vi "Shut Down Device.vi"(8 "error in (no error)":errorcluster, 11 "Power Meter in":refnum<class "Power Meter.lvclass">) -> (0 "error out":errorcluster, 3 "Power Meter out":refnum<class "Power Meter.lvclass">)   [LabVIEW 2018, in "Power Meter.lvlib" / "Power Meter.lvclass"]
uses:
  Power Meter.lvclass
  Power Meter.lvclass/Power Meter.ctl
  Device/Device.lvclass
  Power Meter.lvlib
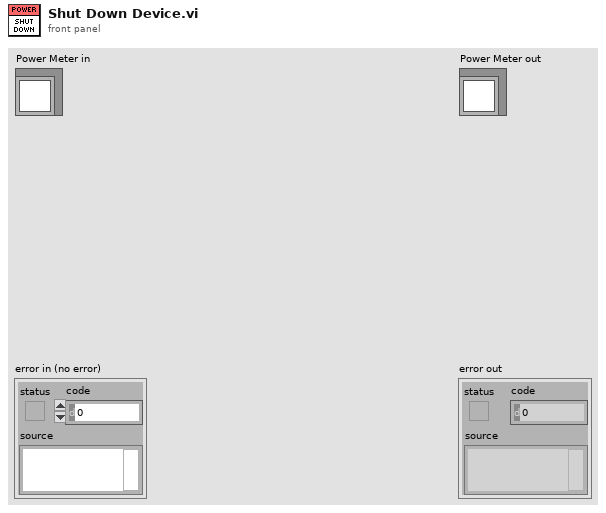
[diagram p1: front panel]
types:
  T1 = enum16{"Disabled", "Thorlabs", "Newport", "Coherent"}
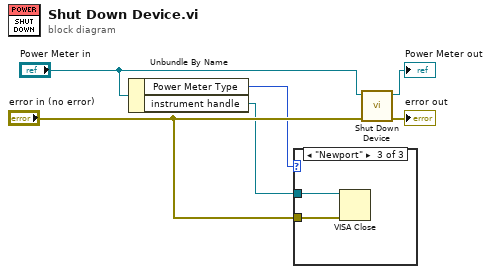
[diagram p0: block diagram]
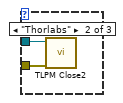
[diagram p3: hidden frame]
diagram:
  n1 = Unbundle By Name("Power Meter in") -> ("Power Meter Type"=w1:T1, "instrument handle"=w2:refnum<visa-resource-name>)
  n2 = case shown="\"Newport\"" w1 {
    tunnel: "error in (no error)" -> [_ w8 w10]
    tunnel: w2 -> [_ w7 w9]
    frame "Disabled", Default {
    }
    frame "Thorlabs" {
      n3 = call "TLPM Close2.vi"("error in (no error)"=w8, "instrument handle"=w7) -> ()  [unwired: 9 in, 1 out]
    }
    frame "Newport" {
      n4 = VISA Close(VISA resource name=w9, error in (no error)=w10) -> ()  [unwired: 1 out]
    }
  }
  n5 = call-parent "Shut Down Device.vi"("error in (no error)"="error in (no error)", "Device in"="Power Meter in") -> ("error out"=→"error out":errorcluster, "Device out"=→"Power Meter out":refnum<class "Power Meter.lvclass">)  [unwired: 8 in]
